vi "Sim_Shoulder.vi"(9 "StartPosDeg":dbl, 11 "Motor Dmd":dbl) -> (1 "MotorRPM":dbl, 2 "Low Limit Switch":bool, 3 "ArmPosDeg":dbl)   [LabVIEW 2023]
uses:
  <vilib>/Rock Robotics/WPI/ThirdParty/JAS_Junk/TrajLib/Enum/DCMOTOR_TYPES_ENUM.ctl
  <vilib>/Rock Robotics/WPI/ThirdParty/JAS_Junk/TrajLib/BatterySim_CalculateLoadedBatteryVoltage.vi
  <vilib>/Rock Robotics/WPI/ThirdParty/JAS_Junk/TrajLib/Trajectory_Library.lvlib
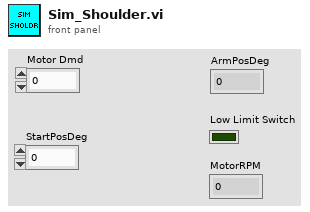
[diagram p1: front panel]
types:
  T1 = typedef "Trajectory_Library.lvlib/DCMOTOR_TYPES_ENUM.ctl" = enum16{"CIM", "AndyMark 9015", "Andy Mark RS 775 125", "Bag", "BaneBots RS 550", "BaneBots RS 775", "Falcon 500", "Mini CIM", "NEO", "NEO 550", "Romi BuiltIn", "Vex 775 Pro", "Snow Blower AM 2235A", "Bosch Seat AM 3493"}
  T2 = typedef "Trajectory_Library.lvlib/LINEAR_SYSTEM_ID_SINGLE_JOINT_ARM_MODEL.ctl" = cluster{"DCMOTOR_TYPES":T1, "Num Motors":i32, "ArmLength_M":dbl, "massKg":dbl, "Gearing":dbl, "MOI kgm2":dbl, "Estimate MOI":bool}
  T3 = typedef "Trajectory_Library.lvlib/SINGLE_JOINT_ARM_SIM_SIMULATION_PARAMS.ctl" = cluster{"MinAngle_Rad":dbl, "MaxAngle_Rad":dbl, "Measurment StdDev":dbl, "SimulateGravity":bool}
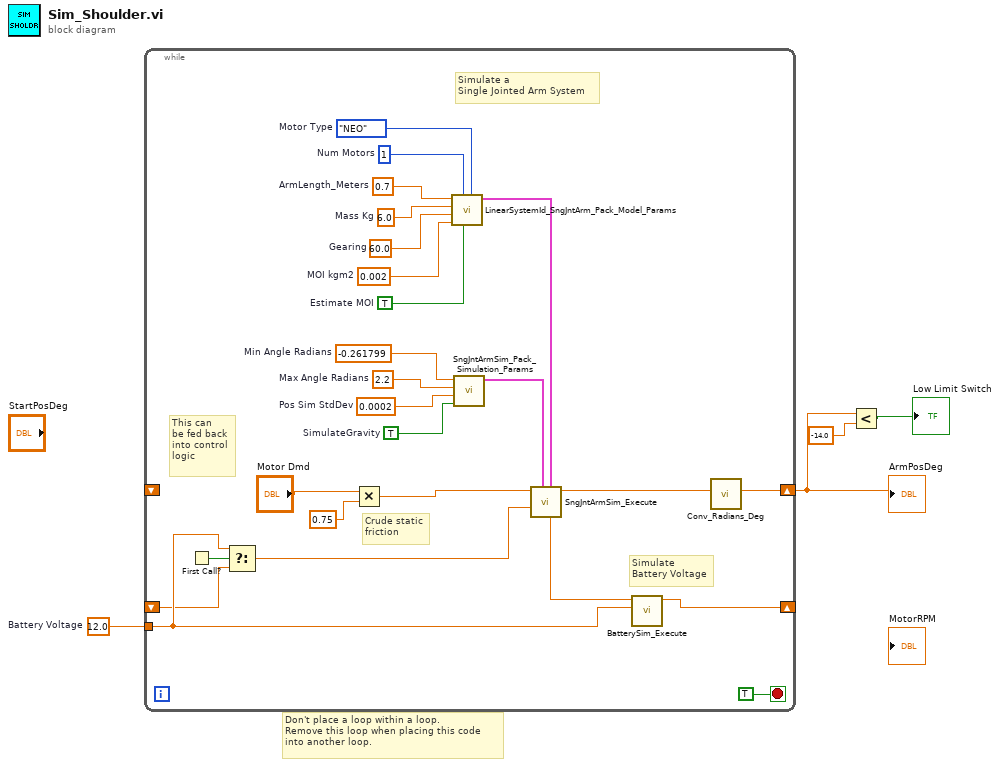
[diagram p0: block diagram]
diagram:
  w4 = 12.0  # Battery Voltage
  # "Don't place a loop within a loop. \nRemove this loop when placing this code\ninto another loop."
  n1 = while {
    shift-right: [w23] -> _
    shift-left: _ -> [w8]
    shift-right: [w5] -> w2
    shift-left: _ -> [_]
    tunnel: w4 -> [w9]
    stop <- TRUE stop-if-true
    w16 = TRUE  # Estimate MOI
    w17 = 0.002  # MOI kgm2
    w18 = -0.261799  # Min Angle Radians
    w19 = 2.2  # Max Angle Radians
    w20 = 0.0002  # Pos Sim StdDev
    w21 = TRUE  # SimulateGravity
    w22 = 0.7  # ArmLength_Meters
    w26 = 60.0  # Gearing
    w27 = 6.0  # Mass Kg
    w28 = 1  # Num Motors
    w29 = DCMOTOR_TYPES_ENUM."NEO"  # Motor Type
    # "Crude static\nfriction"
    # "This can\nbe fed back\ninto control\nlogic"
    # "Simulate\nBattery Voltage"
    # "Simulate a\nSingle Jointed Arm System"
    n2 = First Call?() -> (First Call?: T/F=w10:bool)
    n3 = Select(t=w9, s=w10, f=w8) -> (s? t:f=w7:dbl)
    n4 = Multiply(x="Motor Dmd", y=0.75) -> (x*y=w13:dbl)
    n5 = call <vilib>:"LinearSystemId_SngJntArm_Pack_Model_Params.vi"("DCMOTOR_TYPES"=w29, "Estimate MOI"=w16, "Num Motors"=w28, "MOI kgm2"=w17, "Gearing"=w26, "massKg"=w27, "ArmLength_M"=w22) -> ("SngJntArmSim_Model _Params"=w15:T2)  [unwired: 4 in]
    n6 = call <vilib>:"SngJntArmSim_Pack_Simulation_Params.vi"("SimulateGravity"=w21, "Pos Sim StdDev Rad"=w20, "MaxAngle_Rad"=w19, "MinAngle_Rad"=w18) -> ("SngJntArmSim_Simulation _Params"=w14:T3)  [unwired: 7 in]
    n7 = call <vilib>:"SngJntArmSim_Execute.vi"("SngJntArmSim_Model _Params"=w15, "SngJntArmSim_Simulation _Params"=w14, "Battery Volts"=w7, "Motor Dmd"=w13) -> ("ArmAngle_Rad"=w6:dbl, "Motor Current"=w24:dbl)  [unwired: 2 in, 4 out]
    n8 = call <vilib>:"BatterySim_Execute.vi"("Nominal Battery Voltage"=w9, "Current"=w24) -> ("Voltage"=w23:dbl)  [unwired: 9 in]
    n9 = call <vilib>:"Conv_Radians_Deg.vi"("Radians"=w6) -> ("Degrees"=w5:dbl)  [unwired: 10 in]
  }
  "ArmPosDeg" <- w2
  n10 = Less?(x=w2, y=-14.0) -> (x < y?=→"Low Limit Switch":bool)
